vi "saveImageLocally.vi"(8 "error in (no error)":errorcluster, 9 "Path":path, 10 "ImageString":string, 11 "ImageStreamDecoder in":refnum<class "ImageStreamDecoder.lvclass">) -> (0 "error out":errorcluster, 1 "Path out":path, 3 "ImageStreamDecoder out":refnum<class "ImageStreamDecoder.lvclass">)   [LabVIEW 2011, in "Hardware.lvlib" / "HWControllers.lvlib" / "ImageStreamDecoder.lvclass"]
uses:
  ImageStreamDecoder.lvclass
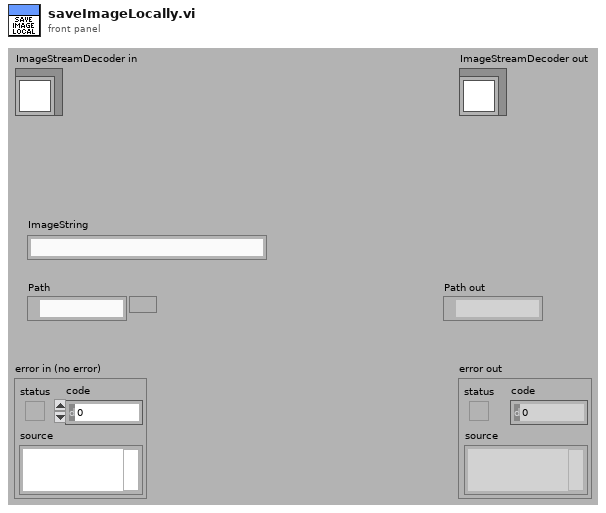
[diagram p1: front panel]
types:
  T1 = typedef "Image Type" = u32
  T2 = typedef "IMAQ Image.ctl" = refnum<image>
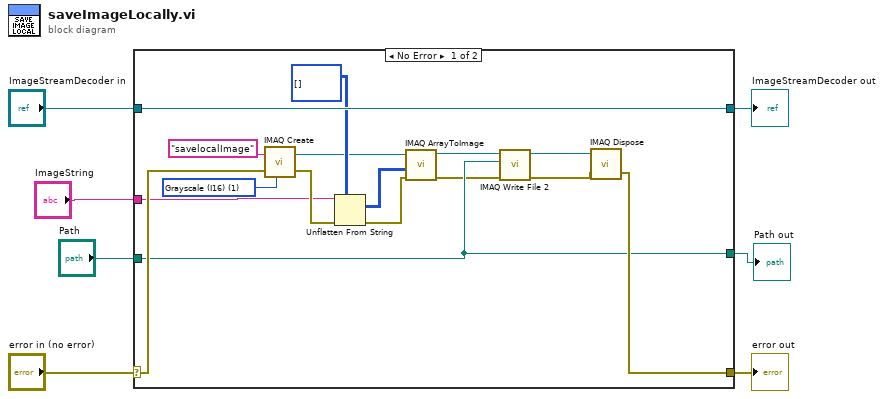
[diagram p0: block diagram]
diagram:
  n1 = case shown="No Error" "error in (no error)" {
    selector: "error in (no error)" -> [w21 w25]
    tunnel: [w15 w25] -> w6
    tunnel: [w23 w24] -> w4
    tunnel: "ImageStreamDecoder in" -> [w23 w24]
    tunnel: "ImageString" -> [w20 _]
    tunnel: "Path" -> [w14 _]
    tunnel: [w14 _] -> w1
    frame No Error {
      w18 = T1 1 items=["Grayscale (U8)", "Grayscale (I16)", "Grayscale (SGL)", "Complex (CSG)", "RGB (U32)", "HSL (U32)", "RGB (U64)", "Grayscale (U16)"] ("Image Type")
      n2 = call "IMAQ Create"("Image Name"="savelocalImage", "Image Type"=w18, "error in (no error)"=w21) -> ("New Image"=w12:T2, "error out"=w22:errorcluster)  [unwired: 2 in]
      n3 = Unflatten From String(type=i16[][] [] ("Image Pixels (I16)"), binary string=w20, error in (no error)=w22) -> (value=w11:i16[][], error out=w8:errorcluster)  [unwired: 2 in, 1 out]
      n4 = call "IMAQ ArrayToImage"("error in (no error)"=w8, "Image Pixels (I16)"=w11, "Image"=w12) -> ("error out"=w9:errorcluster, "Image Out"=w10:T2)  [unwired: 7 in]
      n5 = call-poly "IMAQ Write File 2"("error in (no error)"=w9, "File Path"=w14, "Image"=w10) -> ("error out"=w16:errorcluster, "Image Out (duplicate)"=w17:T2)  [unwired: 7 in]
      n6 = call "IMAQ Dispose"("Image"=w17, "error in (no error)"=w16) -> ("error out"=w15:errorcluster)  [unwired: 4 in]
    }
    frame Error {
    }
  }
  "error out" <- w6
  "ImageStreamDecoder out" <- w4
  "Path out" <- w1
